vi "Actor Core.vi"(8 "error in":errorcluster, 11 "Feedback Dialog in":refnum<class "Feedback Dialog.lvclass">) -> (0 "error out":errorcluster={"status"=TRUE, "code"=1556, "source"="In Place Element Structure in Actor Framework.lvlib:Message Priority Queue.lvclass:Priority Dequeue.vi:2780001->Actor Framework.lvlib:Actor.lvclass:Actor Core.vi:5880001->UI Window.lvlib:UI Window.lvclass:Actor Core.vi:5880001->Feedback Dialog.lvlib:Feedback Dialog.lvclass:Actor Core.vi"}, 3 "Actor out":refnum<class "Actor.lvclass">)   [LabVIEW 2015, in "Feedback Dialog.lvlib" / "Feedback Dialog.lvclass"]
doc: "(<B>Filename</B>: Actor Framework.lvlib:Actor.lvclass:Actor Core.vi)\n\nReceives messages to the actor, reacts to them, and initiates any error handling that may shut the actor down.\n\nDescendant classes may override this VI to append parallel tasks for the actor to complete while it handles messages. Overrides use the Call Parent Method node."
uses:
  Feedback Dialog.lvclass
  UI Window/UI Window.lvclass
  <vilib>/ActorFramework/Stop Msg/Stop Msg.lvclass
  <vilib>/ActorFramework/Actor/Actor.lvclass
panel:
  in  "Cancel Button":bool
  in  "OK Button":bool
  in  "Add Feedback":string
  out "Previous Feedback":string
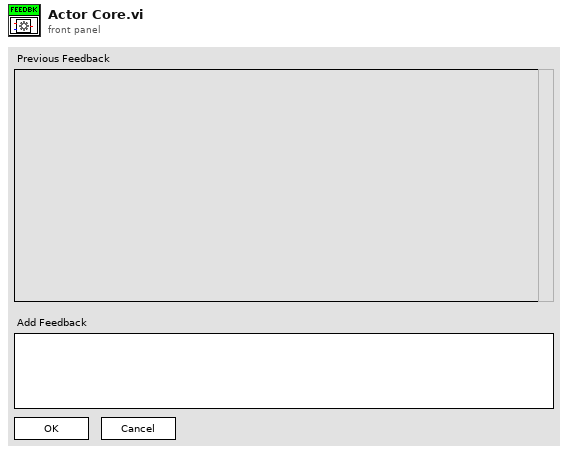
[diagram p1: front panel]
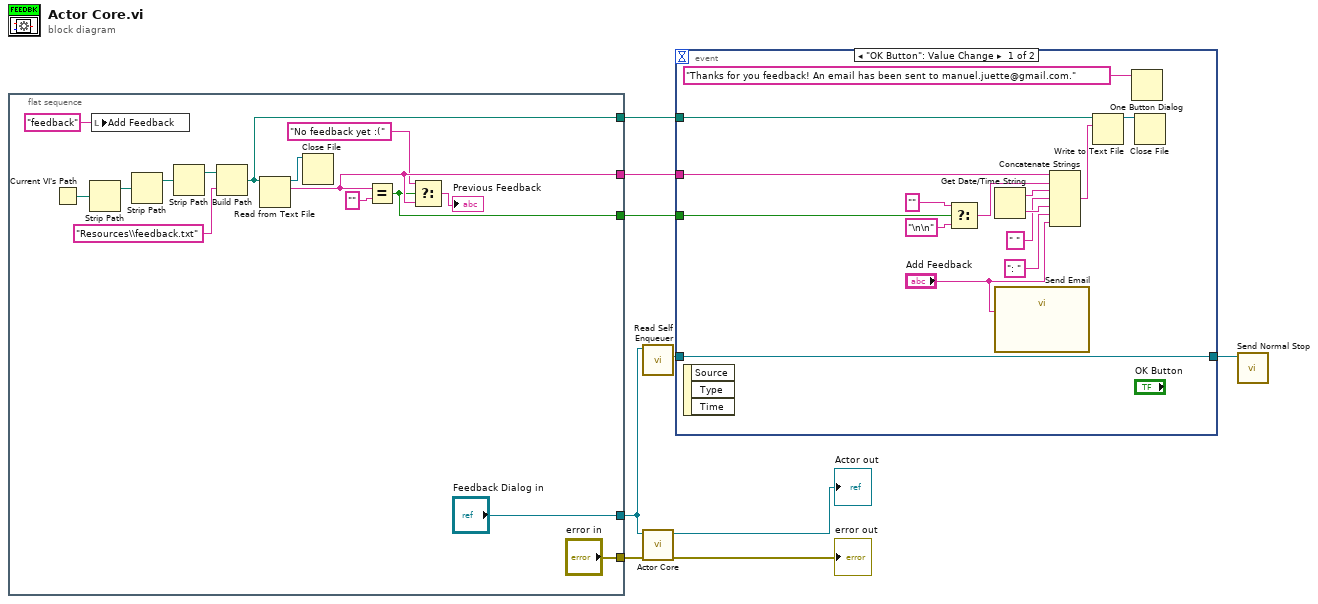
[diagram p0: block diagram]
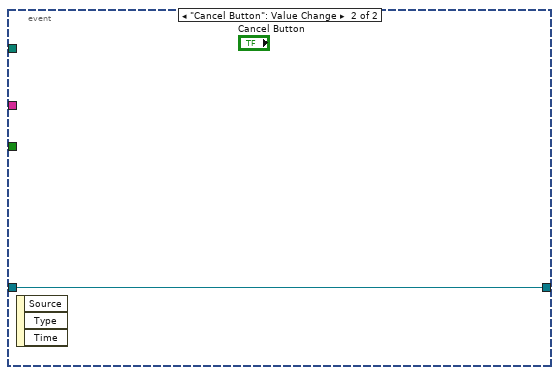
[diagram p2: hidden frame]
diagram:
  n1 = flat-sequence {
    tunnel: ["Feedback Dialog in"] -> w6
    tunnel: ["error in"] -> w7
    tunnel: [w16] -> w3
    tunnel: [w14] -> w2
    tunnel: [w11] -> w1
    frame #0 {
      n2 = Current VI's Path() -> (path=w22:path)
      n3 = Strip Path(path=w22) -> (stripped path=w23:path)  [unwired: 1 out]
      n4 = local write "Add Feedback"("feedback" ("Add Feedback")) -> ()
      n5 = Strip Path(path=w23) -> (stripped path=w21:path)  [unwired: 1 out]
      n6 = Strip Path(path=w21) -> (stripped path=w20:path)  [unwired: 1 out]
      n7 = Build Path(base path=w20, name or relative path="Resources\\feedback.txt") -> (appended path=w16:path)
      n8 = Read from Text File(file (use dialog)=w16) -> (refnum out=w17:refnum<file>, text=w14:string)  [unwired: 3 in, 2 out]
      n9 = Close File(refnum=w17) -> ()  [unwired: 1 in, 2 out]
      n10 = Equal?(x=w14, y="") -> (x = y?=w11:bool)
      n11 = Select(t="No feedback yet :(", s=w11, f=w14) -> (s? t:f=→"Previous Feedback":string)
    }
  }
  n12 = call <vilib>:"Read Self Enqueuer.vi"("Actor"=w6) -> ("Self Enqueuer"=w5:refnum<class "Message Enqueuer.lvclass">)  [unwired: 10 in]
  n13 = call-parent "Actor Core.vi"("error in"=w7, "UI Window in"=w6) -> ("error out"=→"error out":errorcluster, "Actor out"=→"Actor out":refnum<class "Actor.lvclass">)  [unwired: 8 in]
  n14 = event shown="[0] \"OK Button\": Value Change" {
    selector: _ -> [_ _]
    dyn-events: _ -> [_ _]
    timeout: _ -> [_ _]
    tunnel: w5 -> [w39 w40]
    tunnel: [w39 w40] -> w4
    tunnel: w3 -> [w37 _]
    tunnel: w2 -> [w36 _]
    tunnel: w1 -> [w31 _]
    event "OK Button": Value Change {
      n15 = event-data() -> ()  [unwired: 1 in, 3 out]
      n16 = Select(t="", s=w31, f="\n\n" ("string")) -> (s? t:f=w29:string)
      n17 = Get Date/Time String() -> (date string=w33:string, time string=w28:string)  [unwired: 3 in]
      n18 = call "Send Email"("Message"="Add Feedback") -> ()  [unwired: 10 in, 1 out]
      n19 = Concatenate Strings(w36, w29, w33, " " ("string"), w28, ": " ("string"), "Add Feedback") -> (w35:string)
      n20 = Write to Text File(file (use dialog)=w37, text=w35) -> (refnum out=w38:refnum<file>)  [unwired: 2 in, 2 out]
      n21 = One Button Dialog(message="Thanks for you feedback! An email has been sent to manuel.juette@gmail.com.") -> ()  [unwired: 1 in, 1 out]
      n22 = Close File(refnum=w38) -> ()  [unwired: 1 in, 2 out]
    }
    event "Cancel Button": Value Change {
      n23 = event-data() -> ()  [unwired: 1 in, 3 out]
    }
  }
  n24 = call <vilib>:"Send Normal Stop.vi"("Message Enqueuer"=w4) -> ()  [unwired: 10 in, 1 out]
